vi "throughWalls_subVI.vi"(4 "Columns":i32, 6 "Rows":i32, 10 "Next X":i32, 11 "Next Y":i32) -> (2 "Next X":i32, 3 "Next Y":i32)   [LabVIEW 2017]
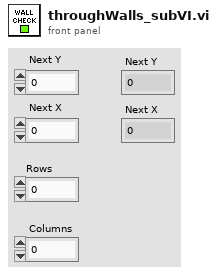
[diagram p1: front panel]
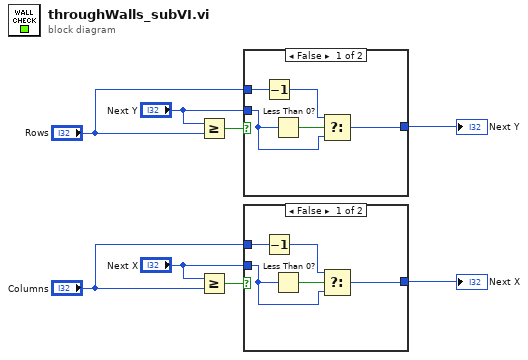
[diagram p0: block diagram]
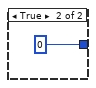
[diagram p2: hidden frame]
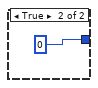
[diagram p3: hidden frame]
diagram:
  n1 = Greater Or Equal?(x="Next Y", y="Rows") -> (x >= y?=w8:bool)
  n2 = Greater Or Equal?(x="Next X", y="Columns") -> (x >= y?=w1:bool)
  n3 = case shown="False" w8 {
    tunnel: [w9 0 ("Next Y")] -> w7
    tunnel: "Next Y" -> [w10 _]
    tunnel: "Rows" -> [w12 _]
    frame False {
      n4 = Decrement(x=w12) -> (x-1=w11:i32)
      n5 = Less Than 0?(x=w10) -> (x < 0?=w13:bool)
      n6 = Select(t=w11, s=w13, f=w10) -> (s? t:f=w9:i32)
    }
    frame True {
    }
  }
  "Next Y" <- w7
  n7 = case shown="False" w1 {
    tunnel: [w15 0 ("Next Y")] -> w2
    tunnel: "Next X" -> [w16 _]
    tunnel: "Columns" -> [w18 _]
    frame False {
      n8 = Decrement(x=w18) -> (x-1=w17:i32)
      n9 = Less Than 0?(x=w16) -> (x < 0?=w19:bool)
      n10 = Select(t=w17, s=w19, f=w16) -> (s? t:f=w15:i32)
    }
    frame True {
    }
  }
  "Next X" <- w2
